vi "DoubleClick.vi"(4 "Point":cluster{"H":T1, "V":T1}, 5 "XRef":refnum<vi>, 6 "State In":T2) -> (0 "Reply":string[](array[string]), 2 "State Out":T2)   [LabVIEW 2012, in "CRefScripting.lvlib" / "CRef Label Node.xnode"]
doc: "This ability VI is called when the user double clicks on your XNode. Point is the the location on the XNode that the user clicked relative to the top-left corner of the XNode. A common pattern is to open a configuration dialog when the user double clicks on an XNode, but you may choose to behave differently. Use Reply to inform LabVIEW of any actions it needs to take.\n\nDefault behavior: None.\n\nThis ability provides UI and OS messages are handled."
uses:
  CRef Label Node.xnode
  State.ctl
  Core/Master Types.ctl
  <vilib>/XNodeSupport/XNodeInt.ctl
  <vilib>/XNodeSupport/NI_XNodeSupport.lvlib
  CRef.lvlib
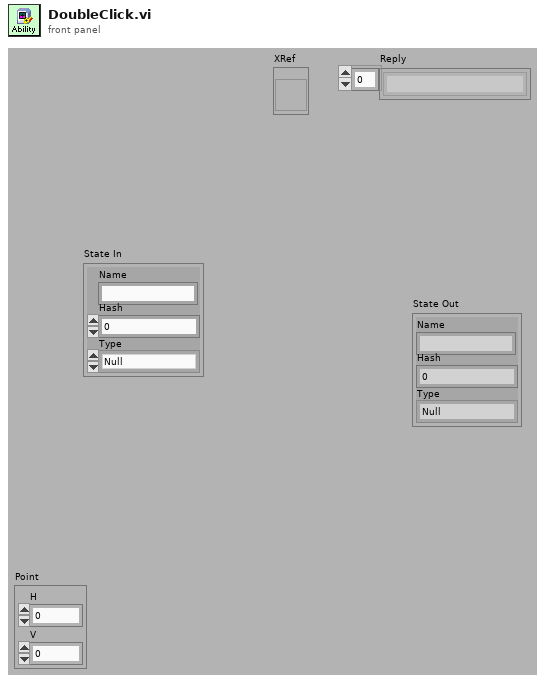
[diagram p1: front panel]
types:
  T1 = typedef "NI_XNodeSupport.lvlib/XNodeInt.ctl" = i32
  T2 = typedef "CRefScripting.lvlib/CRef Label Node.xnode/State.ctl" = cluster{"Name":string, "Hash":u32, "Type":T3}
  T3 = typedef "CRef.lvlib/Master Types.ctl" = enum8{"Null", "Boolean", "U8", "I8", "U16", "I16", "U32", "I32", "U64", "I64", "Single", "Double", "Extended", "CSG", "CDB", "CXT", "Boolean(Def)", "U8(Def)", "I8(Def)", "U16(Def)", "I16(Def)", "U32(Def)", "I32(Def)", "Reserved Def", "Reserved Def1", "Single(Def)", "Double(Def)", "Reserved Def2", "Reserved Def3", "Reserved Def4", "Reserved Def5", "Unsigned(Def)", "Signed(Def)", "Real(Def)", "Reserved Def6", "Numeric(Def)", "String"}
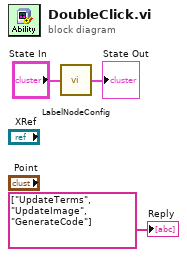
[diagram p0: block diagram]
diagram:
  n1 = call "LabelNodeConfig.vi"("State In"="State In") -> ("State Out"=→"State Out":T2)  [unwired: 3 in, 1 out]
  "Reply" <- string[] ["UpdateTerms", "UpdateImage", "GenerateCode"] ("Reply")
